vi "HCC 2015 Parse.vi"(9 "Fault Set?":bool, 10 "HEWH Appliance Data":string[][](array[string]), 11 "Diagnostic":T1) -> (0 "Basket Speed (RPM) (0xF30B)":i32, 1 "Current RMS (Amps) (0xF30D)":dbl, 2 "Machine Status Color":u32(colorbox), 3 "Cycle Count (0x008E)":i32, 5 "Diagnostic Out":T1)   [LabVIEW 2016]
uses:
  Type Definitions/ViperHawk/ViperHawk Diagnostic Data.ctl
  <vilib>/Utility/error.llb/whitespace.ctl
  Utility/Save File/Global/Save File Globals HCC.vi
panel:
  out "Machine State (0xF10A)":string
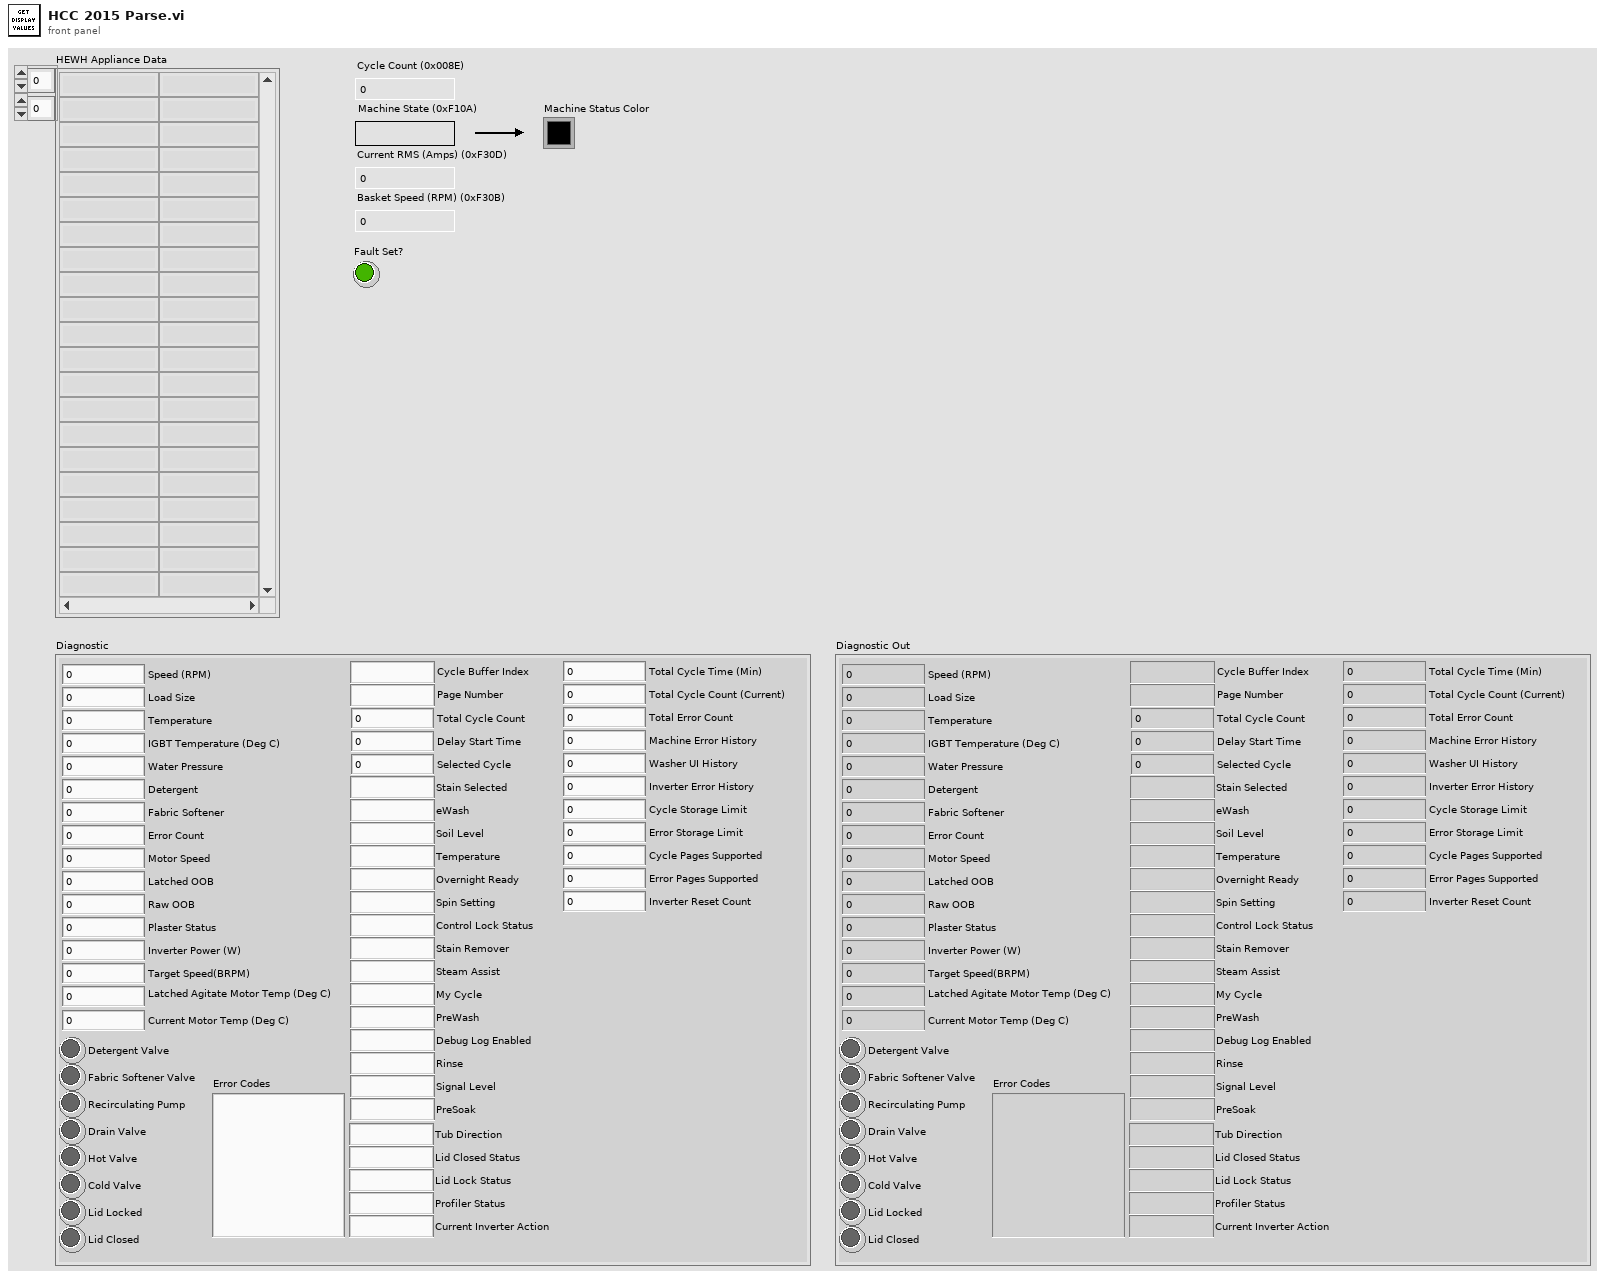
[diagram p1: front panel]
types:
  T1 = typedef "ViperHawk Diagnostic Data.ctl" = cluster{"Speed (RPM)":u32, "Load Size":u32, "Temperature":u32, "Water Pressure":dbl, "Detergent":u32, "Fabric Softener":u32, "Tub Direction":string, "Detergent Valve":bool, "Fabric Softener Valve":bool, "Recirculating Pump":bool, "Drain Valve":bool, "Hot Valve":bool, "Cold Valve":bool, "Lid Closed Status":string, "Lid Lock Status":string, "Error Count":u32, "IGBT Temperature (Deg C)":u32, "Motor Speed":u32, "Latched OOB":u32, "Raw OOB":u32, "Plaster Status":u32, "Inverter Power (W)":u32, "Target Speed(BRPM)":u32, "Latched Agitate Motor Temp (Deg C)":u32, "Current Motor Temp (Deg C)":u32, "Profiler Status":string, "Current Inverter Action":string, "Error Codes":string, "Lid Locked":bool, "Lid Closed":bool, "9E Diagnostic Data":cluster{"Total Cycle Time (Min)":u32, "Total Cycle Count (Current)":u16, "Total Error Count":u16, "Machine Error History":u32, "Washer UI History":u32, "Inverter Error History":u32, "Cycle Storage Limit":u8, "Error Storage Limit":u8, "Cycle Pages Supported":u8, "Error Pages Supported":u8, "Inverter Reset Count":u16}, "9F Diagnostic Data":cluster{"Cycle Buffer Index":string, "Page Number":string, "Total Cycle Count":u32, "Delay Start Time":u32, "Stain Selected":string, "Selected Cycle":u32, "eWash":string, "Soil Level":string, "Temperature":string, "Overnight Ready":string, "Spin Setting":string, "Control Lock Status":string, "Stain Remover":string, "Steam Assist":string, "My Cycle":string, "PreWash":string, "Debug Log Enabled":string, "Rinse":string, "Signal Level":string, "PreSoak":string}}
  T2 = typedef "whitespace.ctl" = u16
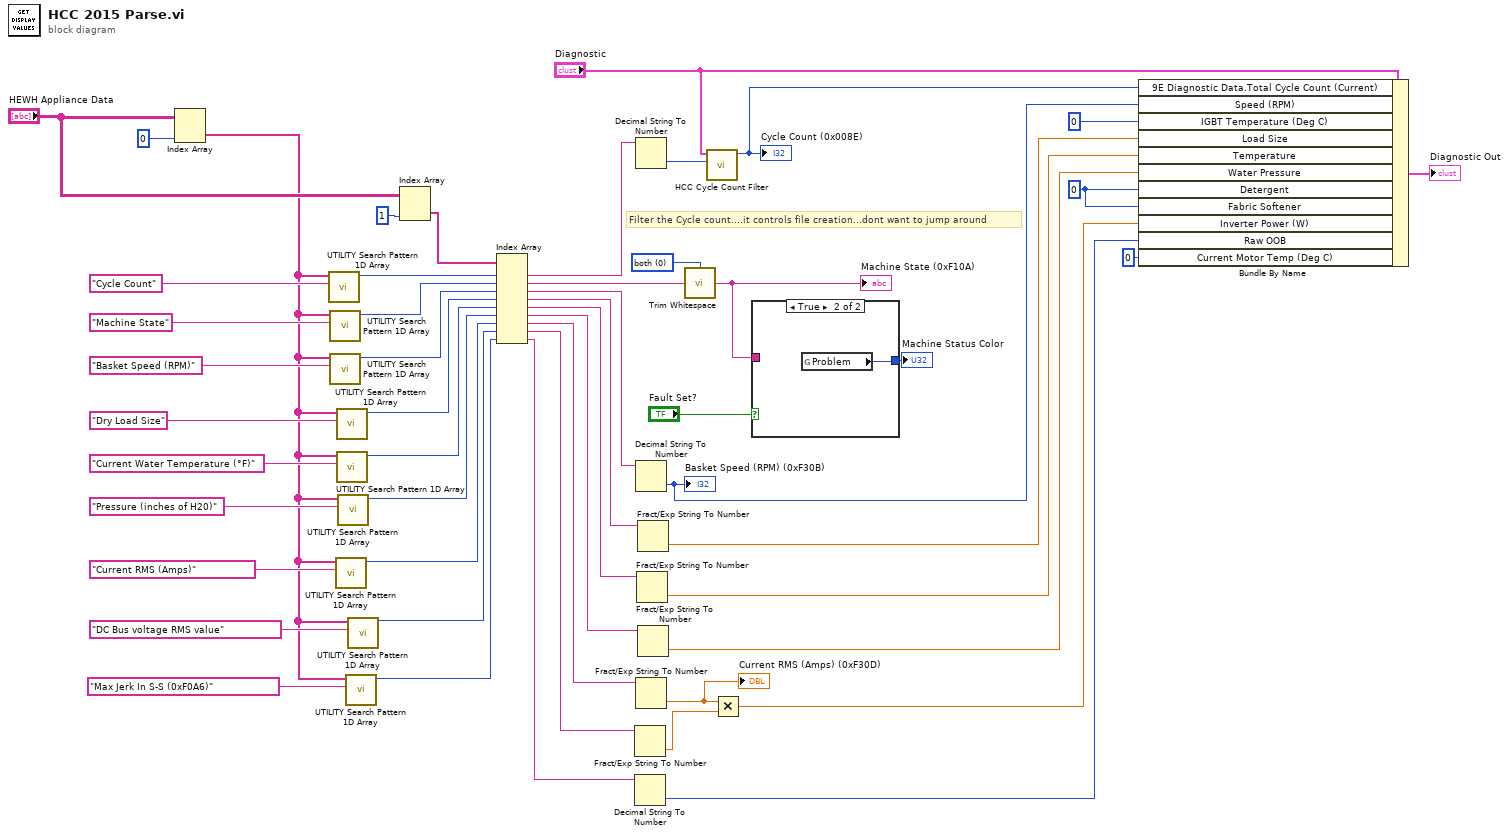
[diagram p0: block diagram]
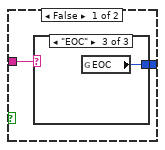
[diagram p2: hidden frame]
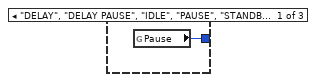
[diagram p3: hidden frame]
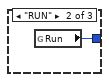
[diagram p4: hidden frame]
diagram:
  w32 = u32 0 ("Detergent")
  w44 = T2 0 items=["both", "start of string", "end of string"] ("location (both)")
  # "Filter the Cycle count....it controls file creation...dont want to jump around"
  n1 = Index Array(array="HEWH Appliance Data", index (col)=0 ("disabled index (col)")) -> (element=w5:string[])  [unwired: 1 in]
  n2 = call "UTILITY Search Pattern 1D Array.vi"("Search Item"="Cycle Count", "1D Array"=w5) -> ("Index"=w21:i32)  [unwired: 9 in]
  n3 = call "UTILITY Search Pattern 1D Array.vi"("Search Item"="Machine State", "1D Array"=w5) -> ("Index"=w19:i32)  [unwired: 9 in]
  n4 = call "UTILITY Search Pattern 1D Array.vi"("Search Item"="Basket Speed (RPM)", "1D Array"=w5) -> ("Index"=w17:i32)  [unwired: 9 in]
  n5 = call "UTILITY Search Pattern 1D Array.vi"("Search Item"="Current RMS (Amps)", "1D Array"=w5) -> ("Index"=w9:i32)  [unwired: 9 in]
  n6 = call "UTILITY Search Pattern 1D Array.vi"("Search Item"="Dry Load Size", "1D Array"=w5) -> ("Index"=w15:i32)  [unwired: 9 in]
  n7 = call "UTILITY Search Pattern 1D Array.vi"("Search Item"="Current Water Temperature (°F)", "1D Array"=w5) -> ("Index"=w13:i32)  [unwired: 9 in]
  n8 = call "UTILITY Search Pattern 1D Array.vi"("Search Item"="Pressure (inches of H20)", "1D Array"=w5) -> ("Index"=w11:i32)  [unwired: 9 in]
  n9 = call "UTILITY Search Pattern 1D Array.vi"("Search Item"="Max Jerk In S-S (0xF0A6)", "1D Array"=w5) -> ("Index"=w4:i32)  [unwired: 9 in]
  n10 = call "UTILITY Search Pattern 1D Array.vi"("Search Item"="DC Bus voltage RMS value", "1D Array"=w5) -> ("Index"=w7:i32)  [unwired: 9 in]
  n11 = Index Array(array="HEWH Appliance Data", index (col)=1 ("disabled index (col)")) -> (element=w48:string[])  [unwired: 1 in]
  n12 = Index Array(array=w48, index #1=w21, index #2=w19, index #3=w17, index #4=w15, index #5=w13, index #6=w11, index #7=w9, index #8=w7, index #9=w4) -> (element #1=w43:string, element #2=w46:string, element #3=w28:string, element #4=w27:string, element #5=w26:string, element #6=w25:string, element #7=w24:string, element #8=w23:string, element #9=w3:string)
  n13 = Fract/Exp String To Number(string=w23) -> (number=w34:dbl)  [unwired: 3 in, 1 out]
  n14 = Decimal String To Number(string=w3) -> (number=w2:i32)  [unwired: 2 in, 1 out]
  n15 = Decimal String To Number(string=w43) -> (number=w42:i32)  [unwired: 2 in, 1 out]
  n16 = Decimal String To Number(string=w28) -> (number=w38:i32)  [unwired: 2 in, 1 out]
  "Basket Speed (RPM) (0xF30B)" <- w38
  n17 = Fract/Exp String To Number(string=w24) -> (number=w29:dbl)  [unwired: 3 in, 1 out]
  "Current RMS (Amps) (0xF30D)" <- w29
  n18 = Fract/Exp String To Number(string=w26) -> (number=w36:dbl)  [unwired: 3 in, 1 out]
  n19 = Fract/Exp String To Number(string=w27) -> (number=w37:dbl)  [unwired: 3 in, 1 out]
  n20 = Fract/Exp String To Number(string=w25) -> (number=w35:dbl)  [unwired: 3 in, 1 out]
  n21 = call <vilib>:"Trim Whitespace.vi"("string"=w46, "location (both)"=w44) -> ("trimmed string"=w45:string)
  "Machine State (0xF10A)" <- w45
  n22 = call "HCC Cycle Count Filter.vi"("Incoming Cycle Count"=w42, "Diagnostic"="Diagnostic") -> ("Filtered Cycle Count"=w39:u16)  [unwired: 7 in, 2 out]
  "Cycle Count (0x008E)" <- w39
  n23 = Multiply(x=w29, y=w34) -> (x*y=w33:dbl)
  n24 = case shown="True" "Fault Set?" {
    tunnel: [w53 w57] -> w47
    tunnel: w45 -> [w52 _]
    frame False {
      n25 = case shown="\"EOC\"" w52 {
        tunnel: [w54 w55 w56] -> w53
        frame "DELAY", "DELAY PAUSE", "IDLE", "PAUSE", "STANDBY", Default {
          n26 = global read "Save File Globals HCC.vi" "Pause"() -> (w54:u32)
        }
        frame "RUN" {
          n27 = global read "Save File Globals HCC.vi" "Run"() -> (w55:u32)
        }
        frame "EOC" {
          n28 = global read "Save File Globals HCC.vi" "EOC"() -> (w56:u32)
        }
      }
    }
    frame True {
      n29 = global read "Save File Globals HCC.vi" "Problem"() -> (w57:u32)
    }
  }
  "Machine Status Color" <- w47
  n30 = Bundle By Name(cluster="Diagnostic", "9E Diagnostic Data.Total Cycle Count (Current)"=w39, "Speed (RPM)"=w38, "IGBT Temperature (Deg C)"=u32 0, "Load Size"=w37, "Temperature"=w36, "Water Pressure"=w35, "Detergent"=w32, "Fabric Softener"=w32, "Inverter Power (W)"=w33, "Raw OOB"=w2, "Current Motor Temp (Deg C)"=u32 0 ("Raw OOB")) -> (→"Diagnostic Out":T1)
